vi "CSM - Internal State Debug Log History.vi"(1 "Length (5000)":i32=5000, 2 "Skip In Runtime? (T)":bool=TRUE, 5 "State":string, 7 "Arguments (\"\")":string, 9 ">> Response Source Message >>":T2, 11 "Source (\"\")":string, 12 "Enable Periodic State Filter? (T)":bool=TRUE, 13 "Settings":T1={"threashold(#/s)"=1.0, "Check Peroid(s)"=2.0}) -> (6 "Debug Log":string)   [LabVIEW 2017, in "Communicable State Machine.lvlib"]
uses:
  Communicable State Machine.lvlib
  _Support/Typedef/_CSM_Response Source Message.ctl
  Utility/Periodic String Filter Setting.ctl
  Utility/_support/Periodic String Filter Level.ctl
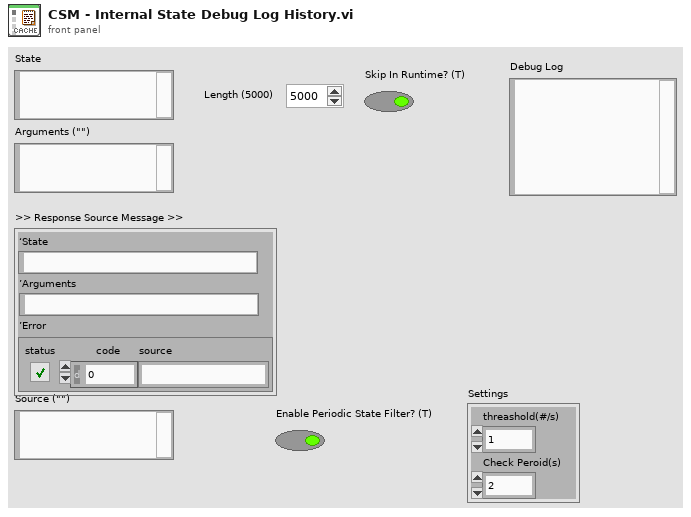
[diagram p1: front panel]
types:
  T1 = typedef "Communicable State Machine.lvlib/Periodic String Filter Setting.ctl" = cluster{"threashold(#/s)":dbl, "Check Peroid(s)":dbl}
  T2 = typedef "Communicable State Machine.lvlib/_CSM_Response Source Message.ctl" = cluster{"‘State":string, "’Arguments":string, "’Error":errorcluster}
  T3 = typedef "Communicable State Machine.lvlib/Periodic String Filter Level.ctl" = enum16{"normal", "L1", "L2", "L3", "L4"}
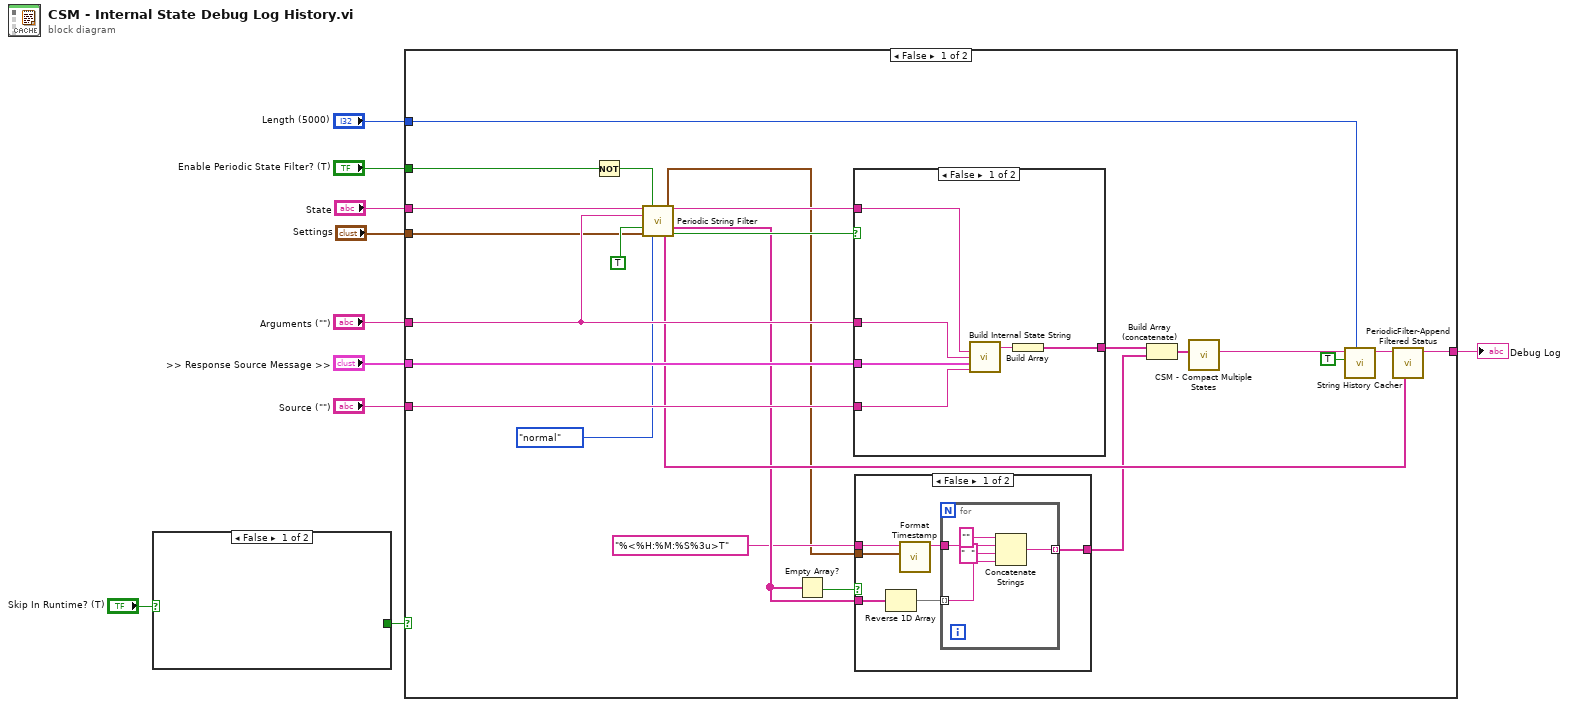
[diagram p0: block diagram]
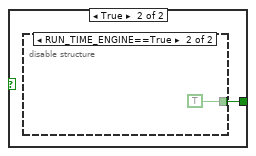
[diagram p2: hidden frame]
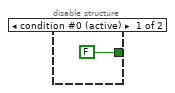
[diagram p3: hidden frame]
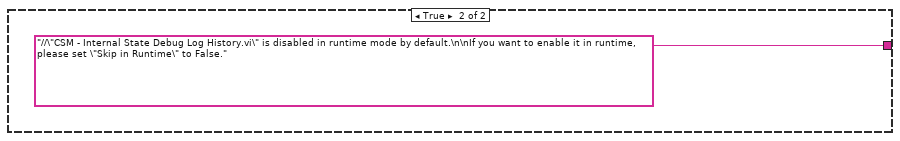
[diagram p6: hidden frame]
diagram:
  n1 = case shown="False" "Skip In Runtime? (T)" {
    tunnel: [_ w11] -> w2
    frame False {
    }
    frame True {
      n2 = disable-structure shown="RUN_TIME_ENGINE==True" {
        disable-tunnel: [FALSE TRUE] -> w11
        frame condition #0 (active) {
        }
        frame condition #1 {
        }
      }
    }
  }
  n3 = case shown="False" w2 {
    tunnel: "Source (\"\")" -> [w37 _]
    tunnel: ">> Response Source Message >>" -> [w36 _]
    tunnel: "State" -> [w35 _]
    tunnel: "Length (5000)" -> [w33 _]
    tunnel: [w23 "//\"CSM - Internal State Debug Log History.vi\" is disabled in runtime mode by default.\n\nIf you want to enable it in runtime, please set \"Skip in Runtime\" to False." ("String Cache")] -> w6
    tunnel: "Enable Periodic State Filter? (T)" -> [w31 _]
    tunnel: "Arguments (\"\")" -> [w29 _]
    tunnel: "Settings" -> [w26 _]
    frame False {
      n4 = Not(x=w31) -> (.not. x?=w28:bool)
      n5 = call "Periodic String Filter.vi"("Input String"=w35, "Reset?"=w28, "Parameter"=w29, "Remove Immediately? (F)"=TRUE ("Remove Immediately?(F)"), "Settings"=w26, "Level (Normal)"=Periodic_String_Filter_Level."normal" ("Level")) -> ("Current Time"=w14:timestamp, "Input String (Dup)"=w32:string, "Additional Info"=w18:string[], "Filtered Status"=w22:string[], "Filtered?"=w27:bool)  [unwired: 5 in]
      n6 = Empty Array?(array=w18) -> (empty?=w19:bool)
      n7 = case shown="False" w27 {
        tunnel: w29 -> [w54 _]
        tunnel: w37 -> [w53 _]
        tunnel: w36 -> [w52 _]
        tunnel: [w49 _] -> w16
        tunnel: w32 -> [w50 _]
        frame False {
          n8 = call "Build Internal State String.vi"("State"=w50, "Arguments (\"\")"=w54, ">> Response Source Message >>"=w52, "Source (\"\")"=w53) -> ("State With Arguments"=w51:string)  [unwired: 11 in]
          n9 = Build Array(w51) -> (w49:string[])
        }
        frame True {
        }
      }
      n10 = case shown="False" w19 {
        tunnel: w14 -> [w43 _]
        tunnel: w18 -> [w42 _]
        tunnel: "%<%H:%M:%S%3u>T" ("Time format string") -> [w41 _]
        tunnel: [w40 _] -> w20
        frame False {
          n11 = Reverse 1D Array(array=w42) -> (reversed array=w38:string[])
          n12 = call "Format Timestamp.vi"("Timestamp"=w43, "Format String"=w41) -> ("String"=w39:string)  [unwired: 9 in]
          n13 = for {
            tunnel: w38 -> [w48] mode=indexing
            tunnel: w39 -> [w45]
            tunnel: [w44] -> w40 mode=indexing
            n14 = Concatenate Strings("" ("string"), w45, "  " ("string"), w48) -> (w44:string)
          }
        }
        frame True {
        }
      }
      n15 = Build Array (concatenate)(w16, w20) -> (w21:string[])
      n16 = call "CSM - Compact Multiple States.vi"("Multiple States"=w21) -> ("States"=w15:string)  [unwired: 9 in]
      n17 = call "String History Cacher.vi"("Length"=w33, "Include Timestamp? (T)"=TRUE ("Include Timestamp(T)"), "String"=w15) -> ("String Cache"=w24:string)  [unwired: 8 in]
      n18 = call "PeriodicFilter-Append Filtered Status.vi"("Filtered Status"=w22, "String Cache In"=w24) -> ("String Cache Out"=w23:string)  [unwired: 9 in]
    }
    frame True {
    }
  }
  "Debug Log" <- w6
